vi "Main.vi"(8 "error":errorcluster, 11 "IsSimulated":bool) -> (0 "Error out":errorcluster)   [LabVIEW 2018, in "IO.lvclass"]
doc: "Use this template to build a simple state machine design pattern. Each state executes code and determines which state to transition to."
uses:
  IO.lvclass
  Controller/Public Controls/GlobalConfig.ctl
  IO.lvclass/IO.ctl
  S1/Public Controls/Outputs.ctl
  S2/Public Controls/Outputs.ctl
  S3/Public Controls/Outputs.ctl
  S4/Public Controls/Outputs.ctl
  S5/Public Controls/Outputs.ctl
  S6/Public Controls/Outputs.ctl
  <vilib>/DAQmx/write.llb/DAQmx Write (Digital Bool 1Line 1Point).vi
  <vilib>/DAQmx/miscellaneous.llb/DAQmx Fill In Error Info.vi
  S1/S1.lvclass
  S2/S2.lvclass
  Controller/GUI.lvclass
  S3/S3.lvclass
  S4/S4.lvclass
  S5/S5.lvclass
  S6/S6.lvclass
panel:
  out "loop":i32
  out "DigitalInput":bool[](array[boolean])
  out "data":waveform(dbl)[](graph)
  # "IO MAIN"
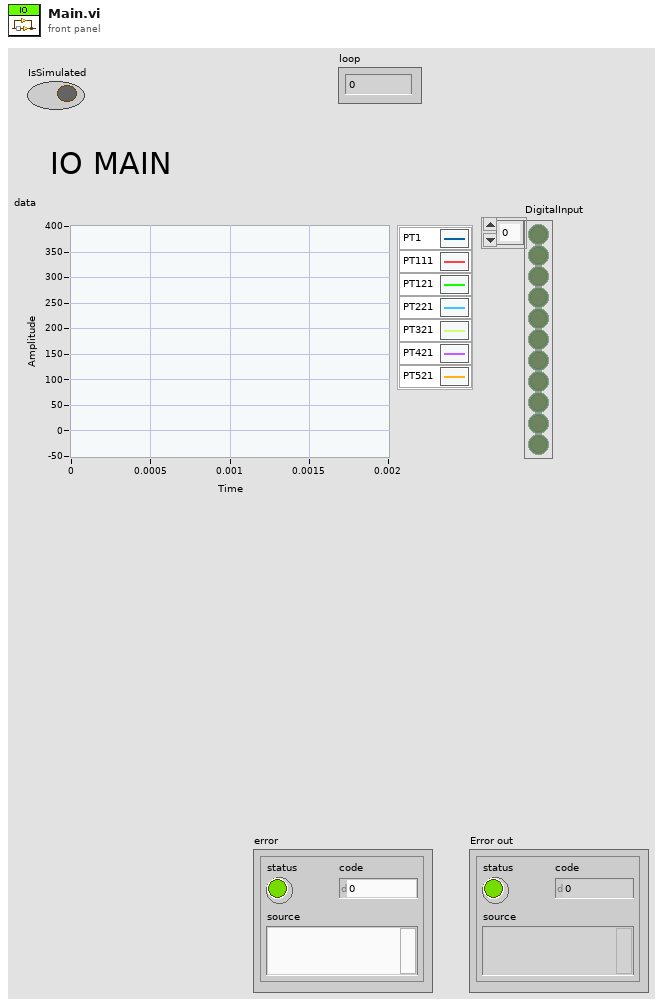
[diagram p1: front panel]
types:
  T1 = typedef "GUI.lvclass/GlobalConfig.ctl" = cluster{"Report Folder Path":path, "PT1_MIN":dbl, "PT1_MAX":dbl, "VENT_PMAX":dbl, "LOP_TARGET":dbl, "LOP_RAMP":dbl, "LOP_LEAK_MAX":dbl, "HIP_TARGET":dbl, "HIP_RAMP":dbl, "HIP_MIN":dbl, "HIP_MAX":dbl, "BLEED_TIME":dbl, "LOP_MAX":dbl, "LOP_MIN":dbl, "PT131Com":refnum<visa-resource-name>, "PT231Com":refnum<visa-resource-name>, "PT331Com":refnum<visa-resource-name>, "PT431Com":refnum<visa-resource-name>, "PT531Com":refnum<visa-resource-name>, "PT631Com":refnum<visa-resource-name>}
  T2 = typedef "S1.lvclass/Outputs.ctl" = cluster{"LoP":bool, "HiP":bool, "Z1Vent":bool, "Z2Vent":bool, "Z3Vent":bool, "IsLidLock":bool}
  T3 = typedef "S2.lvclass/Outputs.ctl" = cluster{"LO P":bool, "HI P":bool, "Z3Vent":bool, "V2 Vent":bool, "IsLidLocked":bool}
  T4 = typedef "S3.lvclass/Outputs.ctl" = cluster{"LO P":bool, "HI P":bool, "Z3Vent":bool, "V2 Vent":bool, "IsLidLocked":bool}
  T5 = typedef "S4.lvclass/Outputs.ctl" = cluster{"LO P":bool, "HI P":bool, "Z3Vent":bool, "V2 Vent":bool, "IsLidLocked":bool}
  T6 = typedef "S5.lvclass/Outputs.ctl" = cluster{"LO P":bool, "HI P":bool, "Z3Vent":bool, "V2 Vent":bool, "IsLidLocked":bool}
  T7 = typedef "S6.lvclass/Outputs.ctl" = cluster{"LO P":bool, "HI P":bool, "Z3Vent":bool, "V2 Vent":bool, "IsLidLocked":bool}
  T8 = typedef "IO.lvclass/State.ctl" = enum16{"Initialize", "GlobalConfig", "ESTOP", "Abort", "S1Ouputs", "S2Outputs", "S3Ouputs", "S4Outputs", "S5Outputs", "S6Outputs", "Read", "Error", "Exit"}
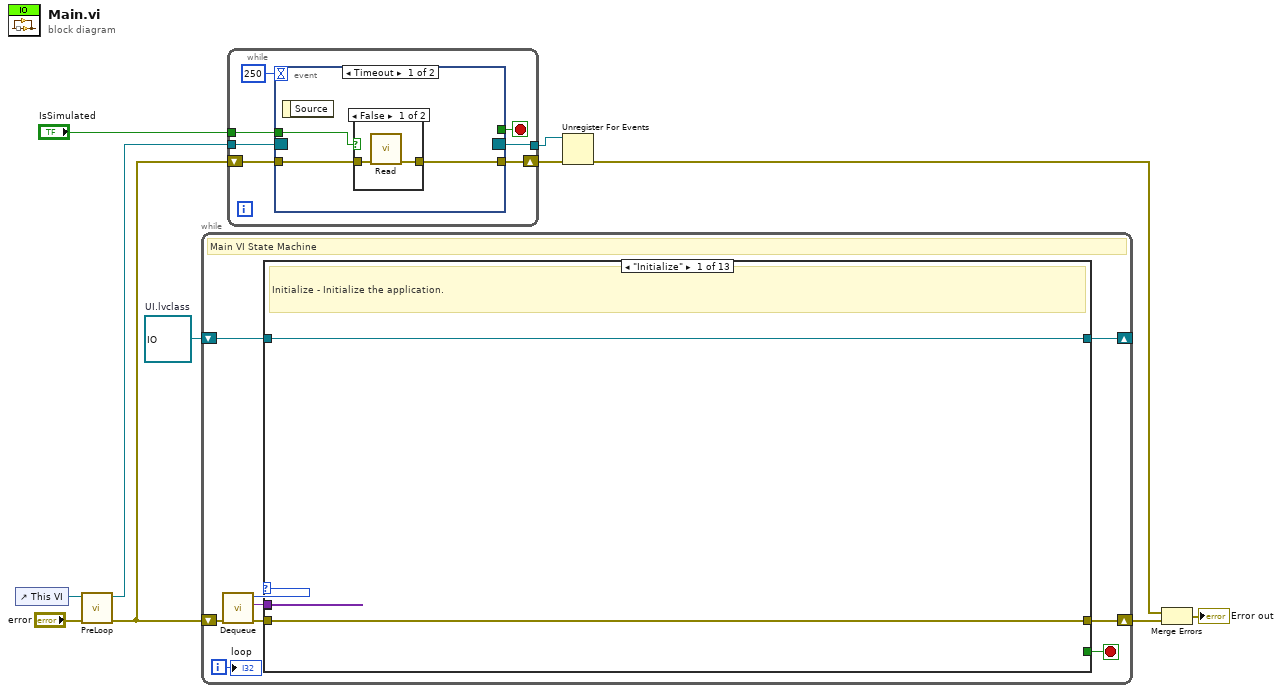
[diagram p0: block diagram]
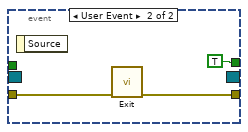
[diagram p3: hidden frame]
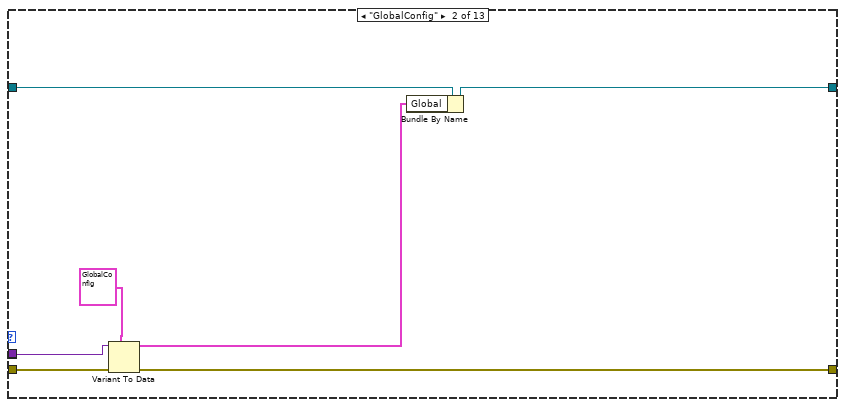
[diagram p4: hidden frame]
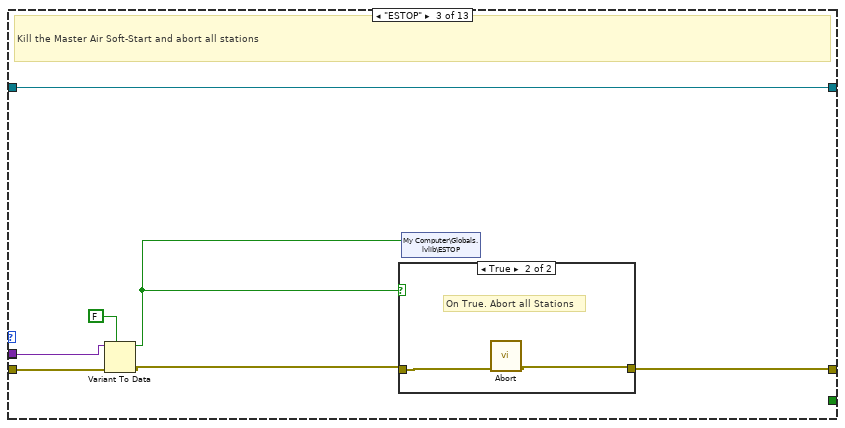
[diagram p5: hidden frame]
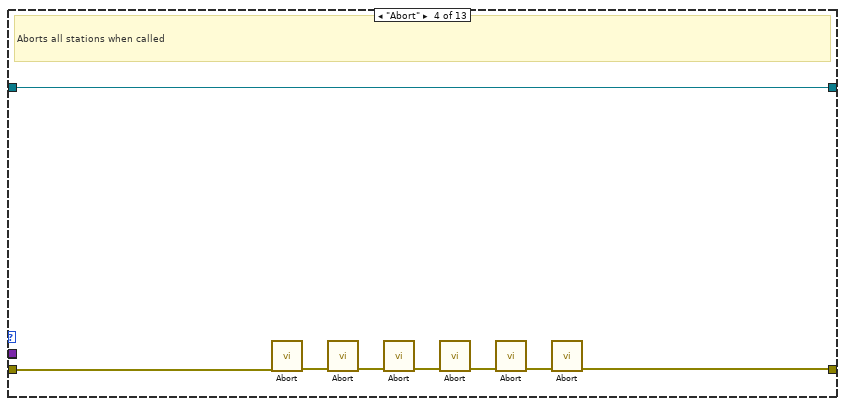
[diagram p7: hidden frame]
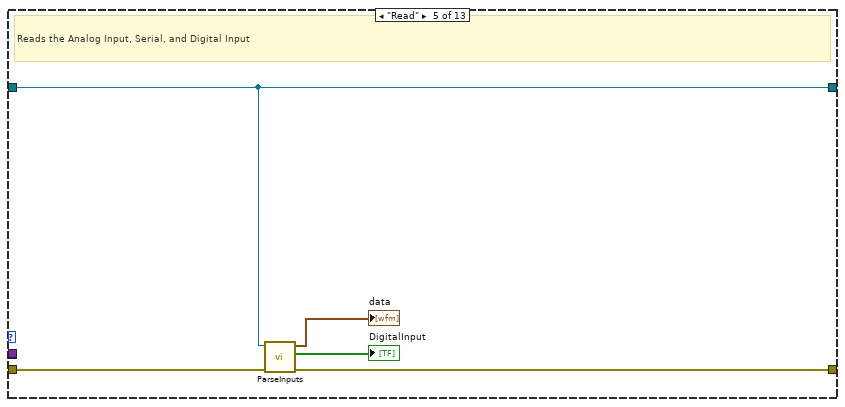
[diagram p8: hidden frame]
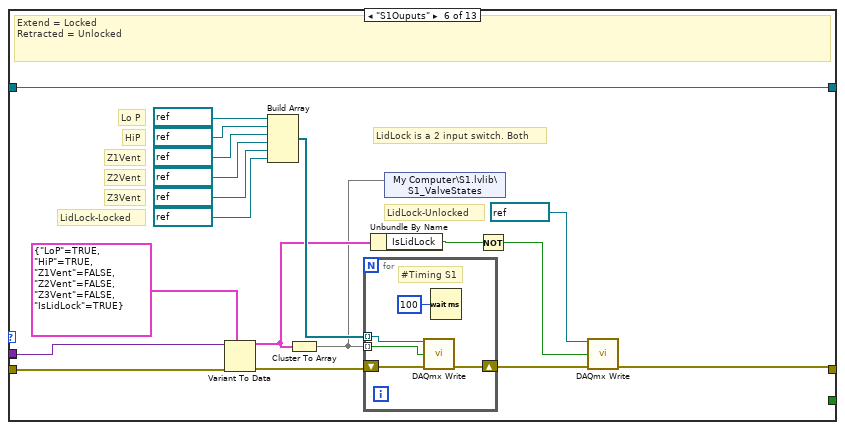
[diagram p9: hidden frame]
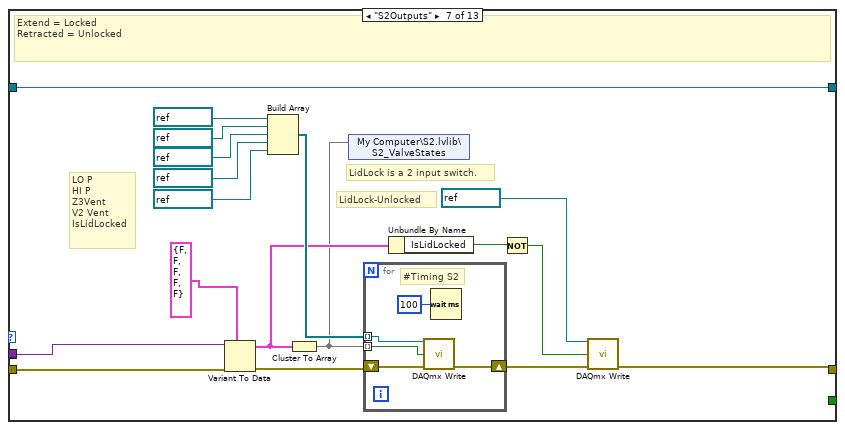
[diagram p10: hidden frame]
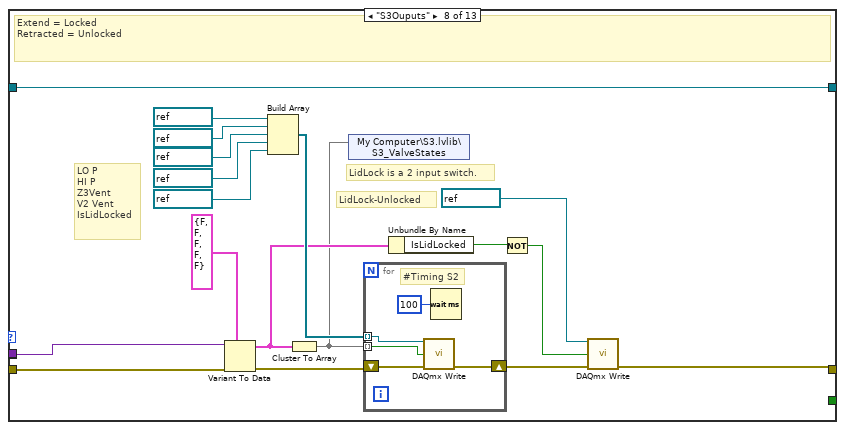
[diagram p11: hidden frame]
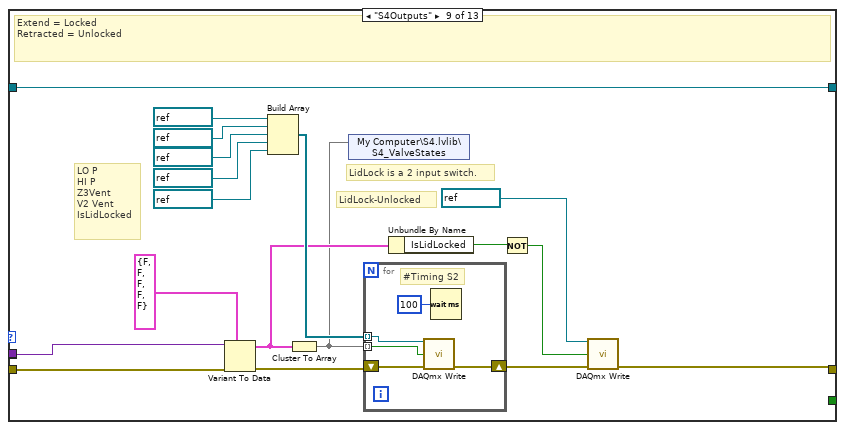
[diagram p12: hidden frame]
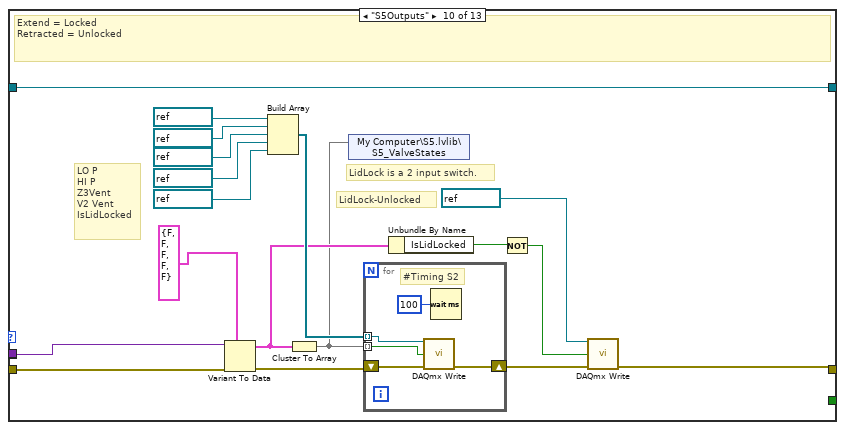
[diagram p13: hidden frame]
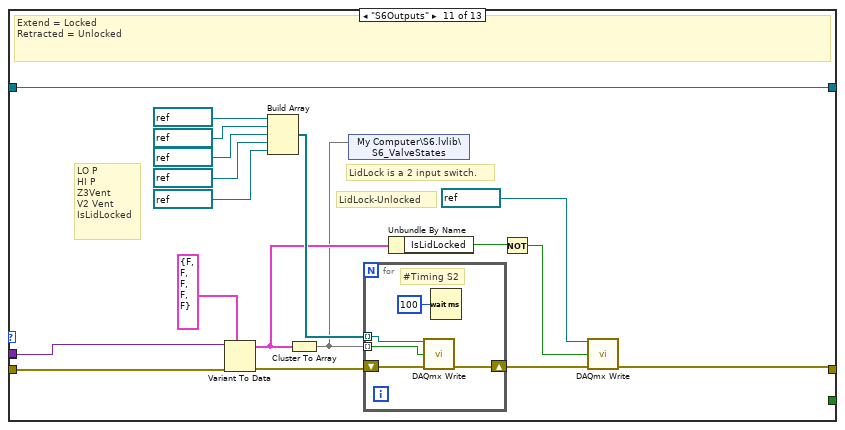
[diagram p14: hidden frame]
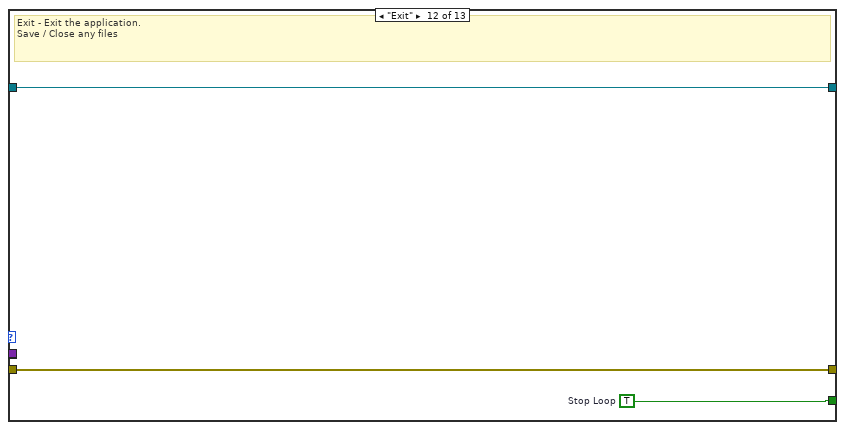
[diagram p15: hidden frame]
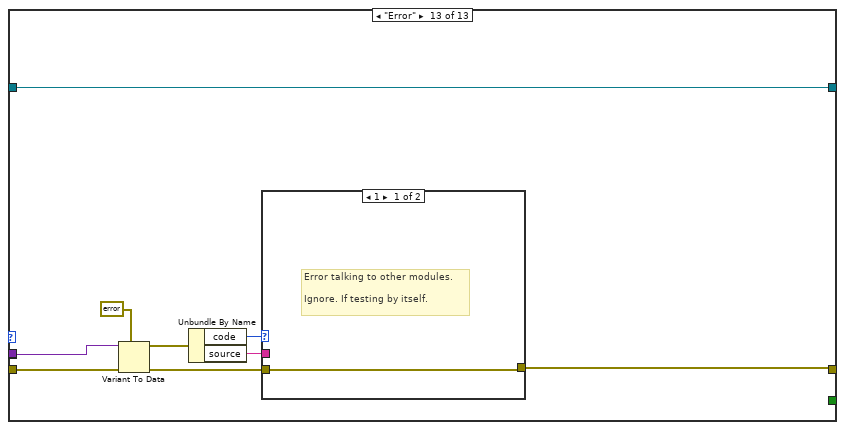
[diagram p16: hidden frame]
diagram:
  w11 = refnum<class "IO.lvclass"> refnum  # UI.lvclass
  n1 = control-ref of="This VI"() -> (w8:refnum<vi>)
  n2 = call "PreLoop.vi"("error in"="error", "VI Ref"=w8) -> ("error out"=w7:errorcluster, "Event Registration Refnum"=w9:refnum<event-registration>)  [unwired: 8 in]
  n3 = while {
    shift-right: [w20] -> w4
    shift-left: w7 -> [w16]
    shift-right: [w17] -> _
    shift-left: w11 -> [w18]
    i -> [w12]
    stop <- w19 stop-if-true
    # "Main VI State Machine"
    n4 = call "Dequeue.vi"("error in"=w16) -> ("error out"=w15:errorcluster, "Data"=w13:variant, "State"=w14:T8)  [unwired: 8 in]
    n5 = case shown="\"Initialize\"" w14 {
      tunnel: [_ _ _ _ _ _ _ _ _ _ _ w194 _] -> w19
      tunnel: w15 -> [w22 w28 w35 w45 w52 w70 w93 w116 w139 w162 w185 w192 w200]
      tunnel: [w22 w23 w31 w40 w51 w55 w82 w105 w128 w151 w174 w192 w196] -> w20
      tunnel: w18 -> [w21 w29 w36 w47 w48 w71 w94 w117 w140 w163 w186 w193 w203]
      tunnel: [w21 w25 w36 w47 w48 w71 w94 w117 w140 w163 w186 w193 w203] -> w17
      tunnel: w13 -> [_ w27 w34 _ _ w69 w92 w115 w138 w161 w184 _ w199]
      tunnel: w13 -> [_ _ _ _ _ _ _ _ _ _ _ _ _]
      frame "Initialize" {
        # "Initialize - Initialize the application."
      }
      frame "GlobalConfig" {
        n6 = Variant To Data(error in=w28, type=T1 {"Report Folder Path"=path "", "PT1_MIN"=0.0, "PT1_MAX"=0.0, "VENT_PMAX"=0.0, "LOP_TARGET"=0.0, "LOP_RAMP"=0.0, "LOP_LEAK_MAX"=0.0, "HIP_TARGET"=0.0, "HIP_RAMP"=0.0, "HIP_MIN"=0.0, "HIP_MAX"=0.0, "BLEED_TIME"=0.0, "LOP_MAX"=0.0, "LOP_MIN"=0.0, "PT131Com"="COM5", "PT231Com"="COM6", "PT331Com"="COM7", "PT431Com"="COM8", "PT531Com"="COM9", "PT631Com"="COM10"} ("Global"), Variant=w27) -> (data=w24:T1, error out=w23:errorcluster)
        n7 = Bundle By Name(cluster=w29, "Global"=w24) -> (w25:refnum<class "IO.lvclass">)
      }
      frame "ESTOP" {
        # "Kill the Master Air Soft-Start and abort all stations"
        n8 = Variant To Data(error in=w35, type=FALSE, Variant=w34) -> (data=w32:bool, error out=w30:errorcluster)
        n9 = case shown="True" w32 {
          tunnel: w30 -> [w37 w39]
          tunnel: [w37 w38] -> w31
          frame False {
          }
          frame True {
            # "On True. Abort all Stations"
            n10 = call "Abort.vi"("error in"=w39) -> ("error out"=w38:errorcluster)  [unwired: 10 in]
          }
        }
        n11 = shared-variable "My Computer\\Globals.lvlib\\ESTOP"(w32) -> ()  [unwired: 1 in, 1 out]
      }
      frame "Abort" {
        # "Aborts all stations when called"
        n12 = call "Abort.vi"("error in"=w45) -> ("error out"=w46:errorcluster)  [unwired: 10 in]
        n13 = call "Abort.vi"("error in"=w46) -> ("error out"=w44:errorcluster)  [unwired: 10 in]
        n14 = call "Abort.vi"("error in"=w44) -> ("error out"=w43:errorcluster)  [unwired: 10 in]
        n15 = call "Abort.vi"("error in"=w43) -> ("error out"=w42:errorcluster)  [unwired: 10 in]
        n16 = call "Abort.vi"("error in"=w42) -> ("error out"=w41:errorcluster)  [unwired: 10 in]
        n17 = call "Abort.vi"("error in"=w41) -> ("error out"=w40:errorcluster)  [unwired: 10 in]
      }
      frame "Read" {
        # "Reads the Analog Input, Serial, and Digital Input"
        n18 = call "ParseInputs.vi"("error in (no error)"=w52, "IO.lvclass"=w48) -> ("error out"=w51:errorcluster, "DigitalInput"=→"DigitalInput":bool[], "data"=→"data":waveform(dbl)[])  [unwired: 7 in]
      }
      frame "S1Ouputs" {
        # "Z3Vent"
        # "Z2Vent"
        # "Z1Vent"
        # "HiP"
        # "Lo P"
        # "LidLock is a 2 input switch. Both"
        # "LidLock-Locked"
        # "LidLock-Unlocked"
        # "Extend = Locked\nRetracted = Unlocked"
        n19 = Variant To Data(error in=w70, type=T2 {"LoP"=TRUE, "HiP"=TRUE, "Z1Vent"=FALSE, "Z2Vent"=FALSE, "Z3Vent"=FALSE, "IsLidLock"=TRUE} ("SIOutputs"), Variant=w69) -> (data=w54:T2, error out=w68:errorcluster)
        n20 = Build Array(refnum<k21> "SV111" ("DAQmx Global Channel"), refnum<k21> "SV112" ("DAQmx Global Channel"), refnum<k21> "SV113" ("DAQmx Global Channel"), refnum<k21> "SV121" ("DAQmx Global Channel"), refnum<k21> "SV131" ("DAQmx Global Channel"), refnum<k21> "SV115" ("DAQmx Global Channel")) -> (w56:refnum<k21>[])
        n21 = Cluster To Array(cluster=w54) -> (array=w53:bool[])
        n22 = for {
          tunnel: w53 -> [w75] mode=indexing
          shift-right: [w74] -> w66
          shift-left: w68 -> [w76]
          tunnel: w56 -> [w73] mode=indexing
          # "#Timing S1"
          n23 = call-poly <vilib>:"DAQmx Write.vi"("task/channels in"=w73, "data"=w75, "error in"=w76) -> ("error out"=w74:errorcluster)  [unwired: 10 in, 2 out]
          n24 = Wait (ms)(milliseconds to wait=u32 100) -> ()  [unwired: 1 out]
        }
        n25 = Unbundle By Name(w54) -> ("IsLidLock"=w65:bool)
        n26 = shared-variable "My Computer\\S1.lvlib\\S1_ValveStates"(w53) -> ()  [unwired: 1 in, 1 out]
        n27 = Not(x=w65) -> (.not. x?=w63:bool)
        n28 = call-poly <vilib>:"DAQmx Write.vi"("task/channels in"=refnum<k21> "SV114" ("DAQmx Global Channel"), "data"=w63, "error in"=w66) -> ("error out"=w55:errorcluster)  [unwired: 10 in, 2 out]
      }
      frame "S2Outputs" {
        # "LO P\nHI P\nZ3Vent\nV2 Vent\nIsLidLocked"
        # "LidLock is a 2 input switch."
        # "LidLock-Unlocked"
        # "Extend = Locked\nRetracted = Unlocked"
        n29 = Variant To Data(error in=w93, type=T3 {"LO P"=FALSE, "HI P"=FALSE, "Z3Vent"=FALSE, "V2 Vent"=FALSE, "IsLidLocked"=FALSE} ("Outputs"), Variant=w92) -> (data=w79:T3, error out=w91:errorcluster)
        n30 = Build Array(refnum<k21> "SV231" ("DAQmx Global Channel"), refnum<k21> "SV232" ("DAQmx Global Channel"), refnum<k21> "SV233" ("DAQmx Global Channel"), refnum<k21> "SV221" ("DAQmx Global Channel"), refnum<k21> "SV215" ("DAQmx Global Channel")) -> (w83:refnum<k21>[])
        n31 = Cluster To Array(cluster=w79) -> (array=w78:bool[])
        n32 = shared-variable "My Computer\\S2.lvlib\\S2_ValveStates"(w78) -> ()  [unwired: 1 in, 1 out]
        n33 = for {
          tunnel: w78 -> [w98] mode=indexing
          shift-right: [w97] -> w90
          shift-left: w91 -> [w99]
          tunnel: w83 -> [w96] mode=indexing
          # "#Timing S2"
          n34 = call-poly <vilib>:"DAQmx Write.vi"("task/channels in"=w96, "data"=w98, "error in"=w99) -> ("error out"=w97:errorcluster)  [unwired: 10 in, 2 out]
          n35 = Wait (ms)(milliseconds to wait=u32 100) -> ()  [unwired: 1 out]
        }
        n36 = Unbundle By Name(w79) -> ("IsLidLocked"=w80:bool)
        n37 = Not(x=w80) -> (.not. x?=w88:bool)
        n38 = call-poly <vilib>:"DAQmx Write.vi"("task/channels in"=refnum<k21> "SV214" ("DAQmx Global Channel"), "data"=w88, "error in"=w90) -> ("error out"=w82:errorcluster)  [unwired: 10 in, 2 out]
      }
      frame "S3Ouputs" {
        # "LO P\nHI P\nZ3Vent\nV2 Vent\nIsLidLocked"
        # "LidLock is a 2 input switch."
        # "LidLock-Unlocked"
        # "Extend = Locked\nRetracted = Unlocked"
        n39 = Variant To Data(error in=w116, type=T4 {"LO P"=FALSE, "HI P"=FALSE, "Z3Vent"=FALSE, "V2 Vent"=FALSE, "IsLidLocked"=FALSE} ("Outputs"), Variant=w115) -> (data=w102:T4, error out=w114:errorcluster)
        n40 = Build Array(refnum<k21> "SV331" ("DAQmx Global Channel"), refnum<k21> "SV332" ("DAQmx Global Channel"), refnum<k21> "SV333" ("DAQmx Global Channel"), refnum<k21> "SV321" ("DAQmx Global Channel"), refnum<k21> "SV315" ("DAQmx Global Channel")) -> (w106:refnum<k21>[])
        n41 = Cluster To Array(cluster=w102) -> (array=w101:bool[])
        n42 = shared-variable "My Computer\\S3.lvlib\\S3_ValveStates"(w101) -> ()  [unwired: 1 in, 1 out]
        n43 = for {
          tunnel: w101 -> [w121] mode=indexing
          shift-right: [w120] -> w113
          shift-left: w114 -> [w122]
          tunnel: w106 -> [w119] mode=indexing
          # "#Timing S2"
          n44 = call-poly <vilib>:"DAQmx Write.vi"("task/channels in"=w119, "data"=w121, "error in"=w122) -> ("error out"=w120:errorcluster)  [unwired: 10 in, 2 out]
          n45 = Wait (ms)(milliseconds to wait=u32 100) -> ()  [unwired: 1 out]
        }
        n46 = Unbundle By Name(w102) -> ("IsLidLocked"=w103:bool)
        n47 = Not(x=w103) -> (.not. x?=w111:bool)
        n48 = call-poly <vilib>:"DAQmx Write.vi"("task/channels in"=refnum<k21> "SV314" ("DAQmx Global Channel"), "data"=w111, "error in"=w113) -> ("error out"=w105:errorcluster)  [unwired: 10 in, 2 out]
      }
      frame "S4Outputs" {
        # "LO P\nHI P\nZ3Vent\nV2 Vent\nIsLidLocked"
        # "LidLock is a 2 input switch."
        # "LidLock-Unlocked"
        # "Extend = Locked\nRetracted = Unlocked"
        n49 = Variant To Data(error in=w139, type=T5 {"LO P"=FALSE, "HI P"=FALSE, "Z3Vent"=FALSE, "V2 Vent"=FALSE, "IsLidLocked"=FALSE} ("Outputs"), Variant=w138) -> (data=w125:T5, error out=w137:errorcluster)
        n50 = Build Array(refnum<k21> "SV431" ("DAQmx Global Channel"), refnum<k21> "SV432" ("DAQmx Global Channel"), refnum<k21> "SV433" ("DAQmx Global Channel"), refnum<k21> "SV421" ("DAQmx Global Channel"), refnum<k21> "SV415" ("DAQmx Global Channel")) -> (w129:refnum<k21>[])
        n51 = Cluster To Array(cluster=w125) -> (array=w124:bool[])
        n52 = shared-variable "My Computer\\S4.lvlib\\S4_ValveStates"(w124) -> ()  [unwired: 1 in, 1 out]
        n53 = for {
          tunnel: w124 -> [w144] mode=indexing
          shift-right: [w143] -> w136
          shift-left: w137 -> [w145]
          tunnel: w129 -> [w142] mode=indexing
          # "#Timing S2"
          n54 = call-poly <vilib>:"DAQmx Write.vi"("task/channels in"=w142, "data"=w144, "error in"=w145) -> ("error out"=w143:errorcluster)  [unwired: 10 in, 2 out]
          n55 = Wait (ms)(milliseconds to wait=u32 100) -> ()  [unwired: 1 out]
        }
        n56 = Unbundle By Name(w125) -> ("IsLidLocked"=w126:bool)
        n57 = Not(x=w126) -> (.not. x?=w134:bool)
        n58 = call-poly <vilib>:"DAQmx Write.vi"("task/channels in"=refnum<k21> "SV414" ("DAQmx Global Channel"), "data"=w134, "error in"=w136) -> ("error out"=w128:errorcluster)  [unwired: 10 in, 2 out]
      }
      frame "S5Outputs" {
        # "LO P\nHI P\nZ3Vent\nV2 Vent\nIsLidLocked"
        # "LidLock is a 2 input switch."
        # "LidLock-Unlocked"
        # "Extend = Locked\nRetracted = Unlocked"
        n59 = Variant To Data(error in=w162, type=T6 {"LO P"=FALSE, "HI P"=FALSE, "Z3Vent"=FALSE, "V2 Vent"=FALSE, "IsLidLocked"=FALSE} ("Outputs"), Variant=w161) -> (data=w148:T6, error out=w160:errorcluster)
        n60 = Build Array(refnum<k21> "SV531" ("DAQmx Global Channel"), refnum<k21> "SV532" ("DAQmx Global Channel"), refnum<k21> "SV533" ("DAQmx Global Channel"), refnum<k21> "SV521" ("DAQmx Global Channel"), refnum<k21> "SV515" ("DAQmx Global Channel")) -> (w152:refnum<k21>[])
        n61 = Cluster To Array(cluster=w148) -> (array=w147:bool[])
        n62 = shared-variable "My Computer\\S5.lvlib\\S5_ValveStates"(w147) -> ()  [unwired: 1 in, 1 out]
        n63 = for {
          tunnel: w147 -> [w167] mode=indexing
          shift-right: [w166] -> w159
          shift-left: w160 -> [w168]
          tunnel: w152 -> [w165] mode=indexing
          # "#Timing S2"
          n64 = call-poly <vilib>:"DAQmx Write.vi"("task/channels in"=w165, "data"=w167, "error in"=w168) -> ("error out"=w166:errorcluster)  [unwired: 10 in, 2 out]
          n65 = Wait (ms)(milliseconds to wait=u32 100) -> ()  [unwired: 1 out]
        }
        n66 = Unbundle By Name(w148) -> ("IsLidLocked"=w149:bool)
        n67 = Not(x=w149) -> (.not. x?=w157:bool)
        n68 = call-poly <vilib>:"DAQmx Write.vi"("task/channels in"=refnum<k21> "SV514" ("DAQmx Global Channel"), "data"=w157, "error in"=w159) -> ("error out"=w151:errorcluster)  [unwired: 10 in, 2 out]
      }
      frame "S6Outputs" {
        # "LO P\nHI P\nZ3Vent\nV2 Vent\nIsLidLocked"
        # "LidLock is a 2 input switch."
        # "LidLock-Unlocked"
        # "Extend = Locked\nRetracted = Unlocked"
        n69 = Variant To Data(error in=w185, type=T7 {"LO P"=FALSE, "HI P"=FALSE, "Z3Vent"=FALSE, "V2 Vent"=FALSE, "IsLidLocked"=FALSE} ("Outputs"), Variant=w184) -> (data=w171:T7, error out=w183:errorcluster)
        n70 = Build Array(refnum<k21> "SV631" ("DAQmx Global Channel"), refnum<k21> "SV632" ("DAQmx Global Channel"), refnum<k21> "SV633" ("DAQmx Global Channel"), refnum<k21> "SV621" ("DAQmx Global Channel"), refnum<k21> "SV615" ("DAQmx Global Channel")) -> (w175:refnum<k21>[])
        n71 = Cluster To Array(cluster=w171) -> (array=w170:bool[])
        n72 = shared-variable "My Computer\\S6.lvlib\\S6_ValveStates"(w170) -> ()  [unwired: 1 in, 1 out]
        n73 = for {
          tunnel: w170 -> [w190] mode=indexing
          shift-right: [w189] -> w182
          shift-left: w183 -> [w191]
          tunnel: w175 -> [w188] mode=indexing
          # "#Timing S2"
          n74 = call-poly <vilib>:"DAQmx Write.vi"("task/channels in"=w188, "data"=w190, "error in"=w191) -> ("error out"=w189:errorcluster)  [unwired: 10 in, 2 out]
          n75 = Wait (ms)(milliseconds to wait=u32 100) -> ()  [unwired: 1 out]
        }
        n76 = Unbundle By Name(w171) -> ("IsLidLocked"=w172:bool)
        n77 = Not(x=w172) -> (.not. x?=w180:bool)
        n78 = call-poly <vilib>:"DAQmx Write.vi"("task/channels in"=refnum<k21> "SV614" ("DAQmx Global Channel"), "data"=w180, "error in"=w182) -> ("error out"=w174:errorcluster)  [unwired: 10 in, 2 out]
      }
      frame "Exit" {
        w194 = TRUE  # Stop Loop
        # "Exit - Exit the application.\nSave / Close any files"
      }
      frame "Error" {
        n79 = Variant To Data(error in=w200, type=errorcluster {"status"=FALSE, "code"=0, "source"=""} ("error out"), Variant=w199) -> (data=w201:errorcluster, error out=w197:errorcluster)
        n80 = Unbundle By Name(w201) -> ("code"=w195:i32, "source"=w198:string)
        n81 = case shown="1" w195 {
          tunnel: w198 -> [_ _]
          tunnel: w197 -> [w204 w205]
          tunnel: [w204 w205] -> w196
          frame 1 {
            # "Error talking to other modules. \n\nIgnore. If testing by itself."
          }
          frame Default {
          }
        }
      }
    }
    "loop" <- w12
  }
  n82 = while {
    tunnel: w9 -> [w207]
    shift-right: [w210] -> w6
    shift-left: w7 -> [w212]
    tunnel: [w209] -> w5
    tunnel: "IsSimulated" -> [w206]
    stop <- w211 stop-if-true
    n83 = event shown="[0] Timeout" {
      selector: w207 -> [_ _]
      dyn-events: [_ _] -> w209
      timeout: 250 -> [_ _]
      tunnel: w212 -> [w215 w221]
      tunnel: [w214 w220] -> w210
      tunnel: [_ TRUE] -> w211
      tunnel: w206 -> [w213 _]
      event Timeout {
        n84 = event-data() -> ()  [unwired: 1 in, 1 out]
        n85 = case shown="False" w213 {
          tunnel: w215 -> [w217 w218]
          tunnel: [w216 w218] -> w214
          frame False {
            n86 = call "Read.vi"("error in"=w217) -> ("error out"=w216:errorcluster)  [unwired: 10 in]
          }
          frame True {
          }
        }
      }
      event User Event {
        n87 = event-data() -> ()  [unwired: 1 in, 1 out]
        n88 = call "Exit.vi"("error in"=w221) -> ("error out"=w220:errorcluster)  [unwired: 10 in]
      }
    }
  }
  n89 = Unregister For Events(event registration refnum=w5, error in=w6) -> (error out=w3:errorcluster)
  n90 = Merge Errors(w3, w4) -> (→"Error out":errorcluster)
